vi "Keithley 27XX Acquire and Graph Time Measurement Data.vi"() -> ()   [LabVIEW 2011]
doc: "This example VI shows how to convert string data elements to numeric elements so it can be graphed and displayed on an XY Graph."
uses:
  Public/Configure/Data/Read Multiple Direct.vi
  Keithley 27XX.lvlib
panel:
  in  "Function (0: DC Voltage)":u16(ring) items=["DC Voltage", "AC Voltage", "DC Current", "AC Current", "Resistance", "Four-Wire Resistance", "Temperature (C)", "Frequency", "Period", "Continuity"]
  in  "Sample Count (10)":i32=10
  in  "Channel List (101:110)":string="101:110"
  out "XY Graph":T1(graph)
  in  "Serial Configuration":T2={"Baud Rate (9600)"=9600, "Flow Control (1: XON/XOFF)"=1, "Termination Char (0:CR)"=0} {"Termination Char (0:CR)" items=["CR", "LF", "CRLF (Do not use)", "LFCR (Do not use)"]; "Flow Control (1: XON/XOFF)" items=["None", "XON/XOFF", "RTS/CTS (2701 Only)", "XON/XOFF & RTS/CTS (2701 Only)"]; "Baud Rate (9600)" items=["300"=300, "600"=600, "1200"=1200, "2400"=2400, "4800"=4800, "9600"=9600, "19.2k"=19200, "38.4k (2701 Only)"=38400, "57.6k (2701 Only)"=57600, "115.2k (2701 Only)"=115200]}
  in  "Timeout (30000 milliseconds)":u32=30000
  in  "VISA resource name":refnum<visa-resource-name>
  # "© 2006 National Instruments Corporation.  ALL RIGHTS RESERVED."
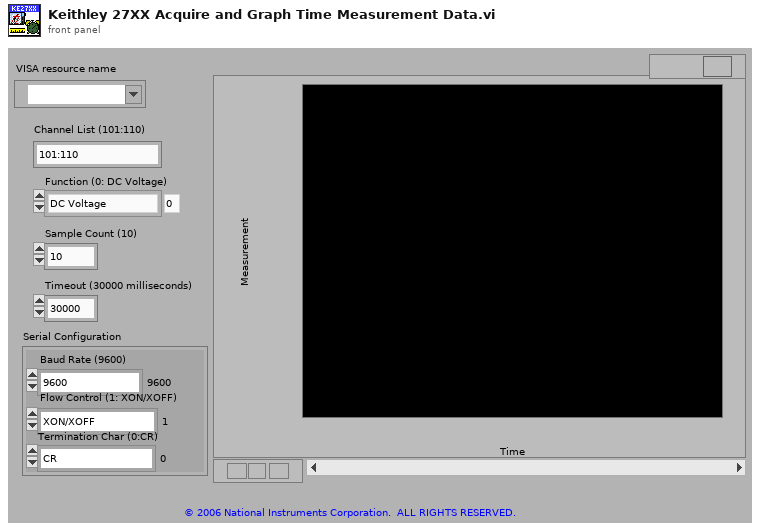
[diagram p1: front panel]
types:
  T1 = cluster{"Measurement Data":dbl[], "Converted Numeric Array":dbl[]}
  T2 = cluster{"Baud Rate (9600)":u32, "Flow Control (1: XON/XOFF)":u16, "Termination Char (0:CR)":u16}
  T3 = cluster{"Numeric Array":dbl[], "Measurement Data":dbl[]}
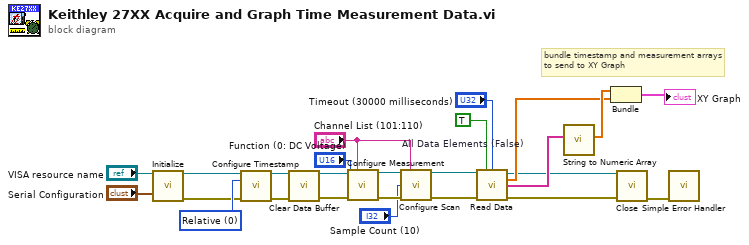
[diagram p0: block diagram]
diagram:
  w12 = u16 0 items=["Relative", "Real Time Clock"] ("Timestamp Type (0: Relative)")
  w23 = TRUE  # All Data Elements (False)
  # "bundle timestamp and measurement arrays to send to XY Graph"
  n1 = call "Initialize.vi"("VISA resource name"="VISA resource name", "Serial Configuration"="Serial Configuration") -> ("VISA resource name out"=w9:refnum<visa-resource-name>, "error out"=w8:errorcluster)  [unwired: 12 in]
  n2 = call "Configure Timestamp.vi"("VISA resource name"=w9, "Timestamp Type (0: Relative)"=w12, "error in (no error)"=w8) -> ("VISA resource name out"=w14:refnum<visa-resource-name>, "error out"=w13:errorcluster)  [unwired: 11 in]
  n3 = call "Clear Data Buffer.vi"("VISA resource name"=w14, "error in (no error)"=w13) -> ("VISA resource name out"=w11:refnum<visa-resource-name>, "error out"=w15:errorcluster)  [unwired: 12 in]
  n4 = call "Configure Measurement.vi"("VISA resource name"=w11, "Scan List (Empty)"="Channel List (101:110)", "Function (0: DC Voltage)"="Function (0: DC Voltage)", "error in (no error)"=w15) -> ("VISA resource name out"=w19:refnum<visa-resource-name>, "error out"=w17:errorcluster)  [unwired: 10 in]
  n5 = call "Configure Scan.vi"("VISA resource name"=w19, "Channel List (101:110)"="Channel List (101:110)", "Sample Count (100)"="Sample Count (10)", "error in (no error)"=w17) -> ("VISA resource name out"=w7:refnum<visa-resource-name>, "error out"=w6:errorcluster)  [unwired: 10 in]
  n6 = call-poly "Read Data.vi"("VISA resource name"=w7, "All Data Elements (False)"=w23, "Timeout (30000 milliseconds)"="Timeout (30000 milliseconds)", "error in (no error)"=w6) -> ("VISA resource name out"=w1:refnum<visa-resource-name>, "Measurement Data"=w3:dbl[], "Time Stamp"=w5:string[], "error out"=w2:errorcluster)  [unwired: 6 in, 2 out]
  n7 = call "String to Numeric Array.vi"("String Array"=w5) -> ("Numeric Array"=w4:dbl[])  [unwired: 10 in]
  n8 = Bundle("Numeric Array"=w4, "Measurement Data"=w3) -> (→"XY Graph":T3)  [unwired: 1 in]
  n9 = call "Close.vi"("VISA resource name"=w1, "error in (no error)"=w2) -> ("error out"=w24:errorcluster)  [unwired: 13 in]
  n10 = call <vilib>:"Simple Error Handler.vi"("error in (no error)"=w24) -> ()  [unwired: 4 in, 5 out]
